vi "ToString.vi"(8 "error in (no error)":errorcluster, 11 "TestCase in":refnum<class "TestCase.lvclass">) -> (0 "error out":errorcluster, 2 "String":string, 3 "TestCase out":refnum<class "TestCase.lvclass">)   [LabVIEW 2019, in "TestCase.lvlib" / "TestCase.lvclass"]
doc: "Returns the string representation for this object."
uses:
  TestCase.lvclass
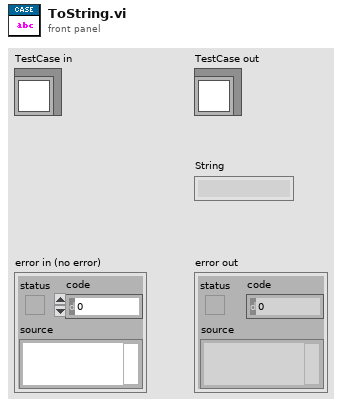
[diagram p1: front panel]
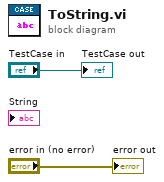
[diagram p0: block diagram]
diagram:
  "error out" <- "error in (no error)"
  "TestCase out" <- "TestCase in"
